vi "Periodic Tasks.vi"(8 "error in":errorcluster) -> ()   [LabVIEW 2013]
doc: "This VI runs in parallel to other tasks. It can contain as many user-defined periodic loops as you need. These can carry out PID or other sorts of timed response."
uses:
  <vilib>/Rock Robotics/SystemInterfaces/Utilities/FPGA_UtilitiesLED Source.ctl
  <vilib>/Rock Robotics/SystemInterfaces/Utilities/FPGA_UtilitiesLED State.ctl
  Robot Global Data.vi
  <vilib>/Rock Robotics/WPI/Compressor/WPI_CompressorGetSetRefNum.vi
  <vilib>/Rock Robotics/WPI/RobotDrive/WPI_RobotDriveGetSetRefNum.vi
  <vilib>/Rock Robotics/WPI/Joystick/WPI_JoystickGetSetRefNum.vi
  Custom VI's/Accelerometer/ADXL345 I2C Axis.ctl
panel:
  out "Distance":dbl
  out "Z":dbl
  out "Y":dbl
  out "X":dbl
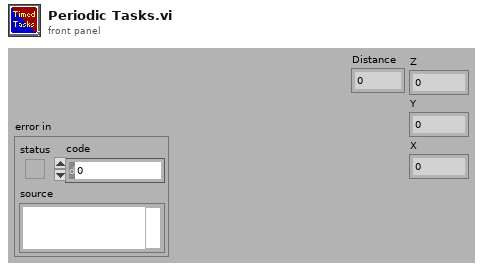
[diagram p1: front panel]
types:
  T1 = typedef "WPI_I2CDevRef.ctl" = cluster{"DevStatus":errorcluster, "Digital Module":T2, "Device Address":u8}
  T2 = typedef "FPGA_TypedefDigitalModule.ctl" = enum16{"Digital Module 1", "Digital Module 2"}
  T3 = typedef "ADXL345 I2C Axis.ctl" = u8
  T4 = typedef "WPI_JoystickDevRef.ctl" = cluster{"Device":T5}
  T5 = typedef "WPI_JoystickDeviceEnum.ctl" = enum16{"USB 1", "USB 2", "USB 3", "USB 4", "Kinect 1", "Kinect 2"}
  T6 = typedef "WPI_RobotDriveDevRef.ctl" = cluster{"DevStatus":errorcluster, "Motors[]":T7[], "Square Inputs":bool, "Max Output":dbl, "Isochronous":bool}
  T7 = typedef "WPI_MotorControlDeviceRef.ctl" = cluster{"DeviceStatus":errorcluster, "Type":enum16{"PWM", "CAN"}, "PWM":cluster{"Digital Module":T2, "PWM Channel":T8, "DeadBand":T9}, "CAN":cluster{"Device Number":u8, "Control Mode":T10, "Semaphore":T11, "Max Vout":dbl}, "Invert":bool, "TransformRef":T12, "InvTransformRef":T12}
  T8 = typedef "FPGA_DIOPWMChannel.ctl" = enum8{"PWM 1", "PWM 2", "PWM 3", "PWM 4", "PWM 5", "PWM 6", "PWM 7", "PWM 8", "PWM 9", "PWM 10", "Invalid"}
  T9 = typedef "WPI_PWMDeadband.ctl" = cluster{"Name":string, "maxPositivePwm":i32, "minPositivePwm":i32, "centerPwm":i32, "maxNegativePwm":i32, "minNegativePwm":i32, "angularRange":u16}
  T10 = typedef "WPI_CANJaguar_ControlMode.ctl" = enum8{"Percent VBus", "Current", "Speed", "Position", "Voltage"}
  T11 = typedef "Semaphore RefNum" = refnum<k1>
  T12 = typedef "WPI_PWMTransform_ConPane.ctl" = refnum<vi>
  T13 = cluster{"JoystickDevRef":T4, "RobotDriveDevRef":T6}
  T14 = typedef "WPI_AnalogChannelDevRef.ctl" = cluster{"DevStatus":errorcluster, "Analog Module":T15, "Analog Channel":T16}
  T15 = typedef "FPGA_TypedefAnalogModule.ctl" = enum16{"Analog Module 1", "Analog Module 2"}
  T16 = typedef "FPGA_AIChannel.ctl" = enum8{"AI 1", "AI 2", "AI 3", "AI 4", "AI 5", "AI 6", "AI 7", "AI 8", "Invalid"}
  T17 = enum16{"Text (00)", "Shoot Status (01)", "Shoot Dist. (02)", "Pressure (03)", "Feed Dist. (04)", "Shutdown (99)"}
  T18 = typedef "FPGA_UtilitiesLED State.ctl" = enum16{"Off", "On", "Toggle"}
  T19 = typedef "FPGA_UtilitiesLED Source.ctl" = enum16{"User LED", "FPGA LED"}
  T20 = typedef "WPI_CompressorDevRef.ctl" = cluster{"DevStatus":errorcluster, "DigitalInputDevRef":T21, "RelayDevRef":T23}
  T21 = typedef "WPI_DigitalInputDevRef.ctl" = cluster{"DevStatus":errorcluster, "DIO Channel":T22, "Digital Module":T2}
  T22 = typedef "FPGA_DIOChannel.ctl" = enum8{"DIO 1", "DIO 2", "DIO 3", "DIO 4", "DIO 5", "DIO 6", "DIO 7", "DIO 8", "DIO 9", "DIO 10", "DIO 11", "DIO 12", "DIO 13", "DIO 14", "Invalid"}
  T23 = typedef "WPI_RelayDevRef.ctl" = cluster{"DevStatus":errorcluster, "Relay Channel":T24, "Digital Module":T2, "Relay Direction":T25}
  T24 = typedef "FPGA_DIORelayChannel.ctl" = enum8{"Relay 1", "Relay 2", "Relay 3", "Relay 4", "Relay 5", "Relay 6", "Relay 7", "Relay 8", "Invalid"}
  T25 = typedef "WPI_RelayDirection.ctl" = enum16{"Both directions", "Forward only", "Reverse only"}
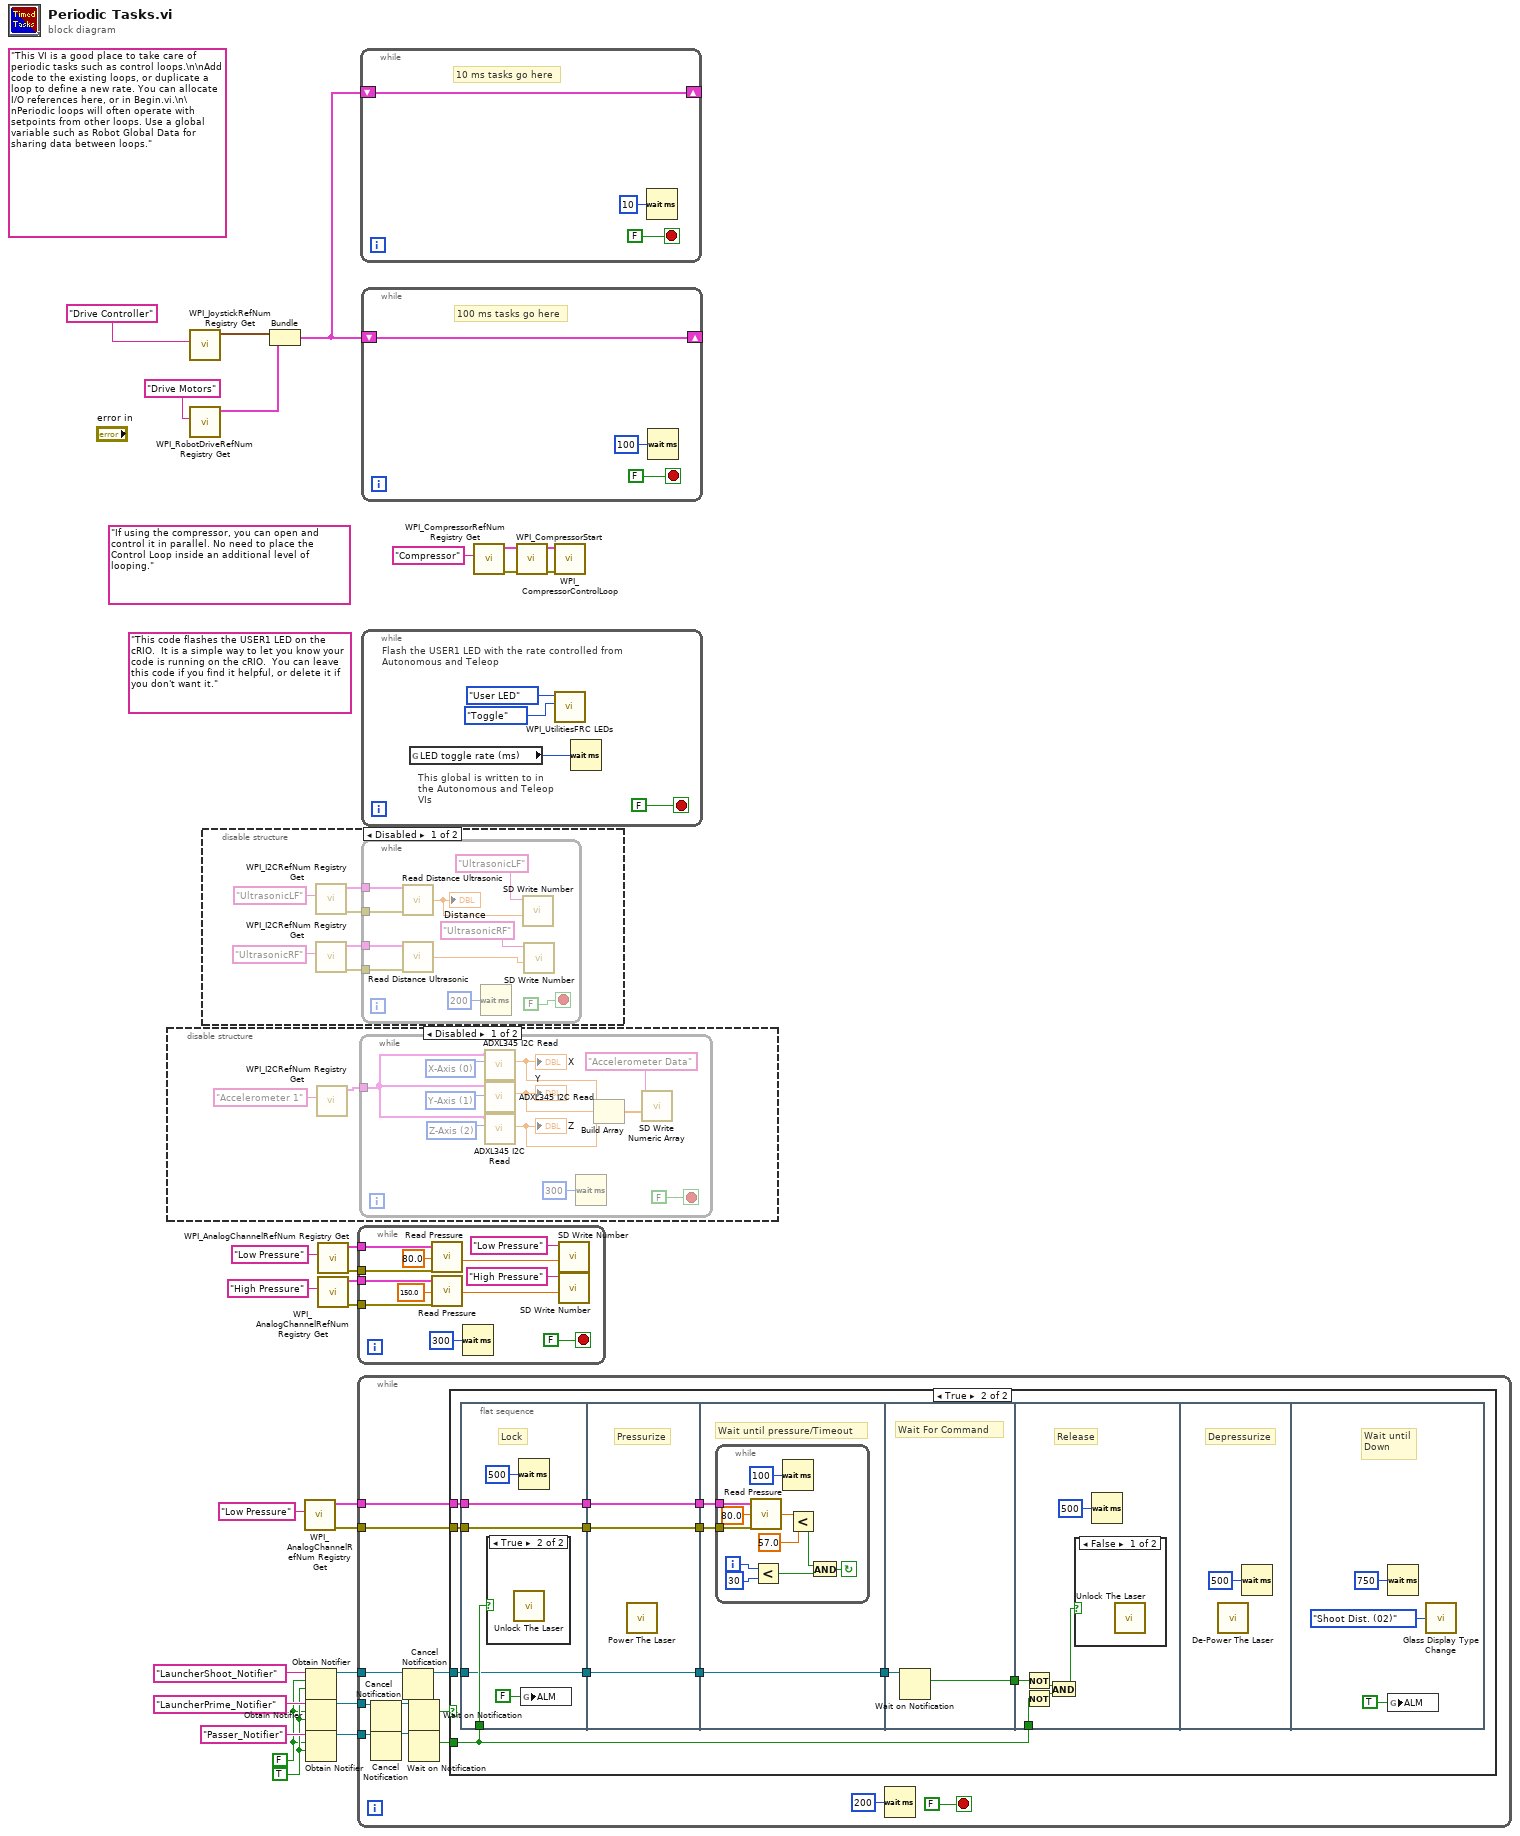
[diagram p0: block diagram]
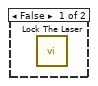
[diagram p4: hidden frame]
diagram:
  w2 = FALSE
  w3 = TRUE ("create if not found? (T)")
  (unwired) "If using the compressor, you can open and control it in parallel. No need to place the Control Loop inside an additional level of looping."
  (unwired) "This code flashes the USER1 LED on the cRIO.  It is a simple way to let you know your code is running on the cRIO.  You can leave this code if you find it helpful, or delete it if you don't want it."
  (unwired) "This VI is a good place to take care of periodic tasks such as control loops.\n\nAdd code to the existing loops, or duplicate a loop to define a new rate. You can allocate I/O references here, or in Begin.vi.\n\nPeriodic loops will often operate with setpoints from other loops. Use a global variable such as Robot Global Data for sharing data between loops."
  n1 = disable-structure shown="Disabled" {
    frame Disabled {
      n2 = call <vilib>:"WPI_I2CRefNum Registry Get.vi"("refnum name"="Accelerometer 1") -> ("I2CDevRef"=w29:T1)  [unwired: 9 in, 1 out]
      n3 = while {
        tunnel: w29 -> [w35]
        stop <- FALSE stop-if-true
        w36 = T3 2 items=["X-Axis", "Y-Axis", "Z-Axis"] ("Axis")
        w37 = T3 1 items=["X-Axis", "Y-Axis", "Z-Axis"] ("Axis")
        w38 = T3 0 items=["X-Axis", "Y-Axis", "Z-Axis"] ("Axis")
        n4 = call "ADXL345 I2C Read.vi"("Axis"=w38, "I2CDevRef"=w35) -> ("Acceleration"=w34:dbl)  [unwired: 7 in, 2 out]
        "X" <- w34
        n5 = call "ADXL345 I2C Read.vi"("Axis"=w37, "I2CDevRef"=w35) -> ("Acceleration"=w33:dbl)  [unwired: 7 in, 2 out]
        "Y" <- w33
        n6 = call "ADXL345 I2C Read.vi"("Axis"=w36, "I2CDevRef"=w35) -> ("Acceleration"=w32:dbl)  [unwired: 7 in, 2 out]
        "Z" <- w32
        n7 = Wait (ms)(milliseconds to wait=u32 300) -> ()  [unwired: 1 out]
        n8 = Build Array(w34, w33, w32) -> (w31:dbl[])
        n9 = call <vilib>:"SD Write Numeric Array.vi"("Numeric Array"=w31, "Name"="Accelerometer Data") -> ()  [unwired: 8 in, 2 out]
      }
    }
    frame Enabled {
    }
  }
  n10 = call <vilib>:"WPI_JoystickRefNum Registry Get.vi"("refnum name"="Drive Controller") -> ("JoystickDevRef"=w25:T4)  [unwired: 1 in, 9 out]
  n11 = call <vilib>:"WPI_RobotDriveRefNum Registry Get.vi"("refnum name"="Drive Motors") -> ("RobotDriveDevRef"=w24:T6)  [unwired: 1 in, 9 out]
  n12 = disable-structure shown="Disabled" {
    frame Disabled {
      n13 = call <vilib>:"WPI_I2CRefNum Registry Get.vi"("refnum name"="UltrasonicLF") -> ("error out"=w44:errorcluster, "I2CDevRef"=w45:T1)  [unwired: 9 in]
      n14 = call <vilib>:"WPI_I2CRefNum Registry Get.vi"("refnum name"="UltrasonicRF") -> ("error out"=w41:errorcluster, "I2CDevRef"=w42:T1)  [unwired: 9 in]
      n15 = while {
        tunnel: w45 -> [w53]
        tunnel: w44 -> [w54]
        tunnel: w42 -> [w50]
        tunnel: w41 -> [w49]
        stop <- FALSE stop-if-true
        n16 = call "Read Distance Ultrasonic.vi"("error out"=w54, "I2CDevRef"=w53) -> ("Inch"=w52:dbl)
        "Distance" <- w52
        n17 = call "Read Distance Ultrasonic.vi"("error out"=w49, "I2CDevRef"=w50) -> ("Inch"=w47:dbl)
        n18 = Wait (ms)(milliseconds to wait=u32 200) -> ()  [unwired: 1 out]
        n19 = call <vilib>:"SD Write Number.vi"("Numeric"=w52, "Name"="UltrasonicLF") -> ()  [unwired: 8 in, 2 out]
        n20 = call <vilib>:"SD Write Number.vi"("Numeric"=w47, "Name"="UltrasonicRF") -> ()  [unwired: 8 in, 2 out]
      }
    }
    frame Enabled {
    }
  }
  n21 = Bundle("JoystickDevRef"=w25, "RobotDriveDevRef"=w24) -> (w23:T13)  [unwired: 1 out]
  n22 = call <vilib>:"WPI_AnalogChannelRefNum Registry Get.vi"("refnum name"="Low Pressure") -> ("error out"=w10:errorcluster, "AIDeviceRef"=w11:T14)  [unwired: 9 in]
  n23 = Obtain Notifier(name (unnamed)="LauncherShoot_Notifier", notification data type=w2, create if not found? (T)=w3) -> (notifier out=w1:refnum<notifier>)  [unwired: 1 in, 2 out]
  n24 = Obtain Notifier(name (unnamed)="LauncherPrime_Notifier", notification data type=w2, create if not found? (T)=w3) -> (notifier out=w7:refnum<notifier>)  [unwired: 1 in, 2 out]
  n25 = Obtain Notifier(name (unnamed)="Passer_Notifier", notification data type=w2, create if not found? (T)=w3) -> (notifier out=w5:refnum<notifier>)  [unwired: 1 in, 2 out]
  n26 = call <vilib>:"WPI_AnalogChannelRefNum Registry Get.vi"("refnum name"="Low Pressure") -> ("error out"=w14:errorcluster, "AIDeviceRef"=w15:T14)  [unwired: 9 in]
  n27 = call <vilib>:"WPI_AnalogChannelRefNum Registry Get.vi"("refnum name"="High Pressure") -> ("error out"=w12:errorcluster, "AIDeviceRef"=w13:T14)  [unwired: 9 in]
  n28 = while {
    tunnel: w15 -> [w66]
    tunnel: w14 -> [w65]
    tunnel: w13 -> [w64]
    tunnel: w12 -> [w63]
    stop <- FALSE stop-if-true
    n29 = call "Read Pressure.vi"("error in (no error)"=w65, "Max Pressure"=80.0, "AIDeviceRef"=w66) -> ("Current Pressure"=w59:dbl)  [unwired: 1 in]
    n30 = call "Read Pressure.vi"("error in (no error)"=w63, "Max Pressure"=150.0, "AIDeviceRef"=w64) -> ("Current Pressure"=w60:dbl)  [unwired: 1 in]
    n31 = Wait (ms)(milliseconds to wait=u32 300) -> ()  [unwired: 1 out]
    n32 = call <vilib>:"SD Write Number.vi"("Numeric"=w59, "Name"="Low Pressure") -> ()  [unwired: 8 in, 2 out]
    n33 = call <vilib>:"SD Write Number.vi"("Numeric"=w60, "Name"="High Pressure") -> ()  [unwired: 8 in, 2 out]
  }
  n34 = while {
    tunnel: w11 -> [w78]
    tunnel: w10 -> [w77]
    tunnel: w7 -> [w72]
    tunnel: w5 -> [w71]
    tunnel: w1 -> [w73]
    stop <- FALSE stop-if-true
    n35 = Cancel Notification(0:w72) -> (8:w69:refnum<notifier>)  [unwired: 1 in, 2 out]
    n36 = Cancel Notification(0:w71) -> (8:w70:refnum<notifier>)  [unwired: 1 in, 2 out]
    n37 = Cancel Notification(0:w73) -> (8:w74:refnum<notifier>)  [unwired: 1 in, 2 out]
    n38 = Wait on Notification(notifier=w69) -> (notification=w76:bool)  [unwired: 3 in, 3 out]
    n39 = Wait on Notification(notifier=w70) -> (notification=w75:bool)  [unwired: 3 in, 3 out]
    n40 = case shown="True" w76 {
      tunnel: w78 -> [_ w90]
      tunnel: w77 -> [_ w89]
      tunnel: w75 -> [_ w86]
      tunnel: w74 -> [_ w82]
      frame False {
      }
      frame True {
        n41 = flat-sequence {
          tunnel: [w98] -> w91
          tunnel: w90 -> [w98]
          tunnel: w89 -> [w97]
          tunnel: [w97] -> w87
          tunnel: w86 -> [w96]
          tunnel: [w95] -> w83
          tunnel: w82 -> [w95]
          tunnel: [w101] -> w92
          tunnel: w91 -> [w101]
          tunnel: [w100] -> w88
          tunnel: w87 -> [w100]
          tunnel: [w99] -> w84
          tunnel: w83 -> [w99]
          tunnel: w92 -> [w104]
          tunnel: w88 -> [w103]
          tunnel: [w102] -> w85
          tunnel: w84 -> [w102]
          tunnel: w85 -> [w117]
          tunnel: [w116] -> w81
          tunnel: w86 -> [w121]
          tunnel: w81 -> [w120]
          frame #0 {
            # "Lock"
            n42 = case shown="True" w96 {
              frame False {
                n43 = call "Lock The Laser.vi"() -> ()  [unwired: 12 in]
              }
              frame True {
                n44 = call "Unlock The Laser.vi"() -> ()  [unwired: 12 in]
              }
            }
            n45 = Wait (ms)(milliseconds to wait=u32 500) -> ()  [unwired: 1 out]
            n46 = global write "Robot Global Data.vi" "ALM"(FALSE ("AAM")) -> ()
          }
          frame #1 {
            # "Pressurize"
            n47 = call "Power The Laser.vi"() -> ()  [unwired: 12 in]
          }
          frame #2 {
            # "Wait until pressure/Timeout"
            n48 = while {
              tunnel: w104 -> [w115]
              tunnel: w103 -> [w114]
              i -> [w109]
              stop <- w107 continue-if-true
              n49 = call "Read Pressure.vi"("error in (no error)"=w114, "Max Pressure"=80.0, "AIDeviceRef"=w115) -> ("Current Pressure"=w112:dbl)  [unwired: 1 in]
              n50 = Less?(x=w109, y=30) -> (x < y?=w105:bool)
              n51 = Wait (ms)(milliseconds to wait=u32 100) -> ()  [unwired: 1 out]
              n52 = Less?(x=w112, y=57.0) -> (x < y?=w106:bool)
              n53 = And(x=w106, y=w105) -> (x .and. y?=w107:bool)
            }
          }
          frame #3 {
            # "Wait For Command"
            n54 = Wait on Notification(notifier=w117) -> (notification=w116:bool)  [unwired: 3 in, 3 out]
          }
          frame #4 {
            # "Release"
            n55 = Not(x=w120) -> (.not. x?=w122:bool)
            n56 = Not(x=w121) -> (.not. x?=w123:bool)
            n57 = And(x=w122, y=w123) -> (x .and. y?=w119:bool)
            n58 = case shown="False" w119 {
              frame False {
                n59 = call "Unlock The Laser.vi"() -> ()  [unwired: 12 in]
              }
              frame True {
              }
            }
            n60 = Wait (ms)(milliseconds to wait=u32 500) -> ()  [unwired: 1 out]
          }
          frame #5 {
            # "Depressurize"
            n61 = call "De-Power The Laser.vi"() -> ()  [unwired: 12 in]
            n62 = Wait (ms)(milliseconds to wait=u32 500) -> ()  [unwired: 1 out]
          }
          frame #6 {
            # "Wait until\nDown"
            n63 = Wait (ms)(milliseconds to wait=u32 750) -> ()  [unwired: 1 out]
            n64 = global write "Robot Global Data.vi" "ALM"(TRUE ("AAM")) -> ()
            n65 = call "Glass Display Type Change.vi"("Data To Glass Type"=T17."Shoot Dist. (02)") -> ()
          }
        }
      }
    }
    n66 = Wait (ms)(milliseconds to wait=u32 200) -> ()  [unwired: 1 out]
  }
  n67 = while {
    shift-right: [w128] -> _
    shift-left: w23 -> [w128]
    stop <- FALSE stop-if-true
    # "10 ms tasks go here"
    n68 = Wait (ms)(milliseconds to wait=u32 10) -> ()  [unwired: 1 out]
  }
  n69 = while {
    shift-right: [w131] -> _
    shift-left: w23 -> [w131]
    stop <- FALSE stop-if-true
    # "100 ms tasks go here"
    n70 = Wait (ms)(milliseconds to wait=u32 100) -> ()  [unwired: 1 out]
  }
  n71 = while {
    stop <- FALSE stop-if-true
    # "This global is written to in the Autonomous and Teleop VIs"
    # "Flash the USER1 LED with the rate controlled from Autonomous and Teleop"
    n72 = global read "Robot Global Data.vi" "LED toggle rate (ms)"() -> (w134:u32)
    n73 = call <vilib>:"WPI_UtilitiesFRC LEDs.vi"("State"=FPGA_UtilitiesLED_State."Toggle", "LED Type"=FPGA_UtilitiesLED_Source."User LED") -> ()  [unwired: 1 in, 9 out]
    n74 = Wait (ms)(milliseconds to wait=w134) -> ()  [unwired: 1 out]
  }
  n75 = call <vilib>:"WPI_CompressorRefNum Registry Get.vi"("refnum name"="Compressor") -> ("error out"=w22:errorcluster, "CompressorDevRef"=w21:T20)  [unwired: 9 in]
  n76 = call <vilib>:"WPI_CompressorStart.vi"("error in (no error)"=w22, "CompressorDevRef"=w21) -> ("error out"=w20:errorcluster, "CompressorDevRef"=w19:T20)  [unwired: 8 in]
  n77 = call <vilib>:"WPI_CompressorControlLoop.vi"("error in (no error)"=w20, "CompressorDevRef"=w19) -> ()  [unwired: 10 in]
